vi "Check Selection.vi"(10 "Ctl Refnum":refnum<vi>) -> (1 "Is VGUI Control":bool, 2 "VGUI Control":refnum<vi>)   [LabVIEW 2020, in "VolatusGUIEditor.lvlib" / "Editor.lvclass"]
uses:
  Editor.lvclass
  897095f8-9e8c-4e04-9e74-99ca68895d41.vi
  Editor.lvclass/Editor.ctl
  VolatusGUIControls/VolatusGUIControls.lvlib
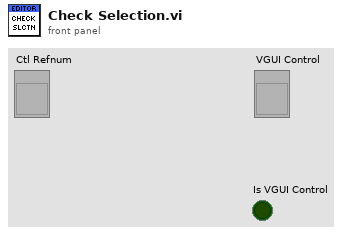
[diagram p1: front panel]
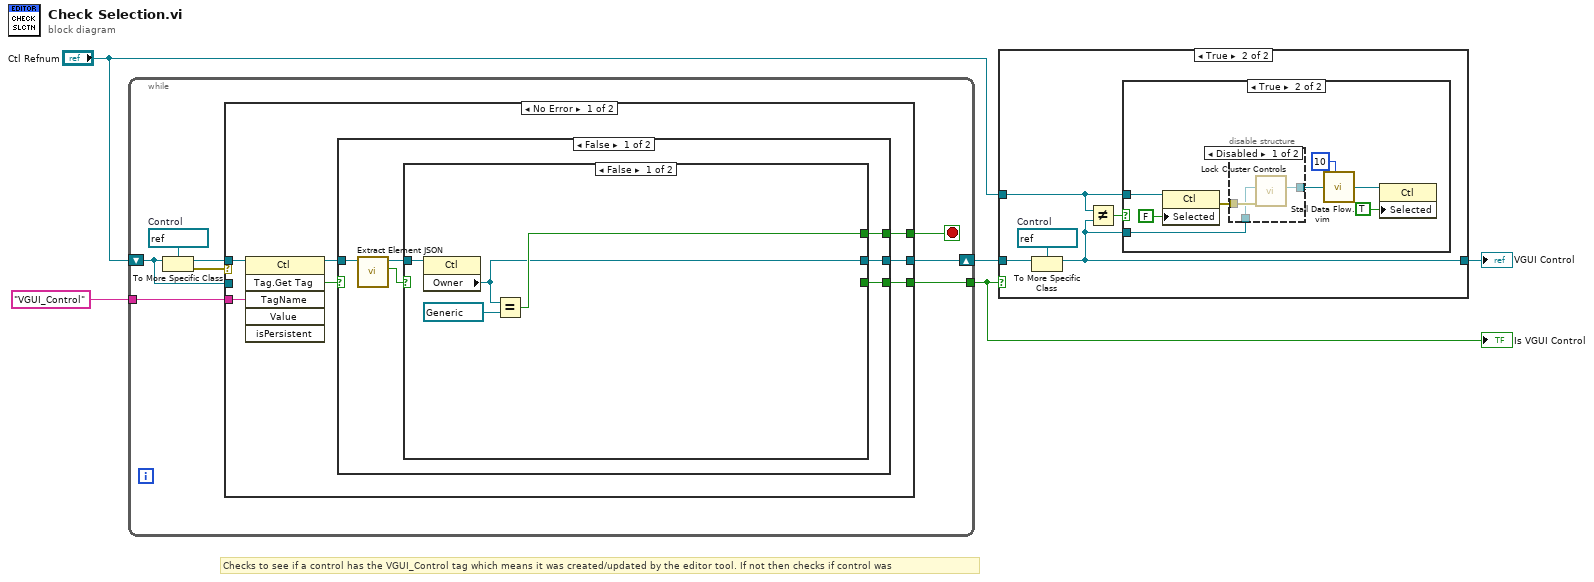
[diagram p0: block diagram]
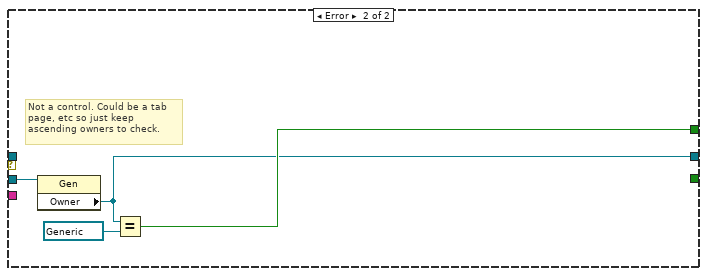
[diagram p7: hidden frame]
diagram:
  # "Checks to see if a control has the VGUI_Control tag which means it was created/updated by the editor tool. If not then checks if control was"
  n1 = while {
    shift-right: [w10] -> w4
    shift-left: "Ctl Refnum" -> [w6]
    tunnel: [w12] -> w3
    tunnel: "VGUI_Control" ("Tag Name") -> [w13]
    stop <- w11 stop-if-true
    w8 = refnum<vi> refnum  # Control
    n2 = To More Specific Class(target class=w8, reference=w6) -> (specific class reference=w9:refnum<vi>, error out=w7:errorcluster)  [unwired: 1 in]
    n3 = case shown="No Error" w7 {
      tunnel: w13 -> [w20 _]
      tunnel: [w18 _] -> w12
      tunnel: [w17 w36] -> w11
      tunnel: [w16 w35] -> w10
      tunnel: w9 -> [w14 _]
      tunnel: w6 -> [_ w38]
      frame No Error {
        n4 = invoke class="Ctl" method="Tag.Get Tag"(reference=w14, "TagName"=w20) -> (reference out=w15:refnum<vi>, "GetTag"=w19:bool)  [unwired: 4 in, 4 out]
        n5 = case shown="False" w19 {
          selector: w19 -> [_ w34]
          tunnel: [w23 w34] -> w18
          tunnel: [w22 w34] -> w17
          tunnel: [w21 w33] -> w16
          tunnel: w15 -> [w26 w33]
          frame False {
            n6 = call "Extract Element JSON.vi"("Ctl Refnum in"=w26) -> ("Is GUI Element"=w24:bool, "Ctl Refnum"=w25:refnum<vi>)  [unwired: 7 in, 2 out]
            n7 = case shown="False" w24 {
              selector: w24 -> [_ w32]
              tunnel: w25 -> [w30 w31]
              tunnel: [_ w32] -> w23
              tunnel: [w28 w32] -> w22
              tunnel: [w27 w31] -> w21
              frame False {
                n8 = property class="Ctl"(reference=w30) -> ("Owner"=w27:refnum<vi>)  [unwired: 1 in, 2 out]
                n9 = Equal?(x=w27, y=refnum<vi> refnum) -> (x = y?=w28:bool)
              }
              frame True {
              }
            }
          }
          frame True {
          }
        }
      }
      frame Error {
        # "Not a control. Could be a tab page, etc so just keep ascending owners to check."
        n10 = property class="Gen"(reference=w38) -> ("Owner"=w35:refnum<vi>)  [unwired: 1 in, 2 out]
        n11 = Equal?(x=w35, y=refnum<vi> refnum) -> (x = y?=w36:bool)
      }
    }
  }
  "Is VGUI Control" <- w3
  n12 = case shown="True" w3 {
    tunnel: w4 -> [_ w43]
    tunnel: "Ctl Refnum" -> [w39 w40]
    tunnel: [w39 w41] -> w1
    frame False {
    }
    frame True {
      w44 = refnum<vi> refnum  # Control
      n13 = To More Specific Class(target class=w44, reference=w43) -> (specific class reference=w41:refnum<vi>)  [unwired: 1 in, 1 out]
      n14 = Not Equal?(x=w40, y=w41) -> (x != y?=w42:bool)
      n15 = case shown="True" w42 {
        tunnel: w41 -> [_ w48]
        tunnel: w40 -> [_ w51]
        frame False {
        }
        frame True {
          n16 = property class="Ctl"(reference=w51, "Selected"=FALSE) -> (error out=w52:errorcluster)  [unwired: 1 in, 1 out]
          n17 = disable-structure shown="Disabled" {
            disable-tunnel: w52 -> [w55 _]
            disable-tunnel: w48 -> [w54 w56]
            disable-tunnel: [w53 w56] -> w47
            frame Disabled {
              n18 = call "Lock Cluster Controls.vi"("error in (no error)"=w55, "Ctl Refnum in"=w54) -> ("Ctl Refnum"=w53:refnum<vi>)  [unwired: 8 in, 1 out]
            }
            frame Enabled {
            }
          }
          n19 = call "Stall Data Flow.vim"("value in"=w47, "milliseconds to wait"=u32 10) -> ("value out"=w46:refnum<vi>)  [unwired: 1 out]
          n20 = property class="Ctl"(reference=w46, "Selected"=TRUE) -> ()  [unwired: 1 in, 2 out]
        }
      }
    }
  }
  "VGUI Control" <- w1
